vi "Save Patterns to Library.vi"(8 "error in (no error)":errorcluster, 11 "MultiPattern Matcher in":refnum<class "MultiPattern Matcher.lvclass">) -> (0 "error out":errorcluster, 3 "MultiPattern Matcher out":refnum<class "MultiPattern Matcher.lvclass">)   [LabVIEW 2013, in "MultiPattern Matcher.lvclass"]
uses:
  MultiPattern Matcher.lvclass
  MultiPattern Matcher.lvclass/MultiPattern Matcher.ctl
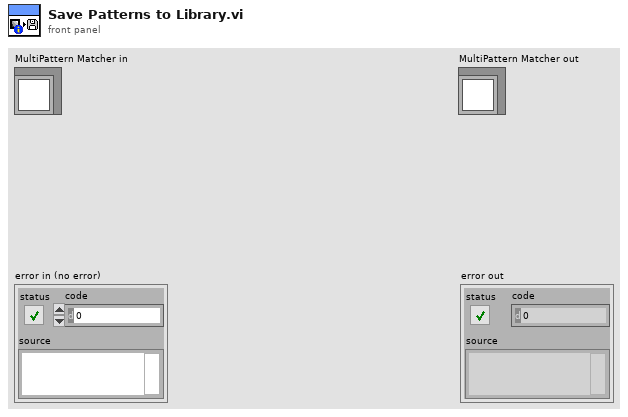
[diagram p1: front panel]
types:
  T1 = typedef "IMAQ Image.ctl" = refnum<image>
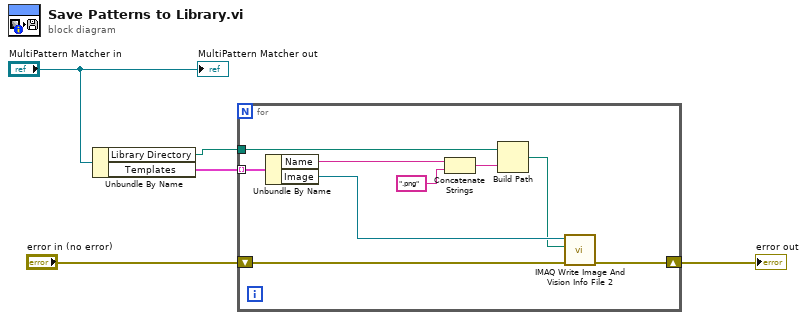
[diagram p0: block diagram]
diagram:
  n1 = Unbundle By Name("MultiPattern Matcher in") -> ("Library Directory"=w3:path, "Templates"=w4:cluster{"Image":T1, "Name":string}[])
  n2 = for {
    shift-right: [w6] -> w2
    shift-left: "error in (no error)" -> [w14]
    tunnel: w4 -> [w13] mode=indexing
    tunnel: w3 -> [w9]
    n3 = Unbundle By Name(w13) -> ("Name"=w11:string, "Image"=w8:T1)
    n4 = Concatenate Strings(w11, ".png" ("string")) -> (w10:string)
    n5 = Build Path(base path=w9, name or relative path=w10) -> (appended path=w7:path)
    n6 = call "IMAQ Write Image And Vision Info File 2"("error in (no error)"=w14, "File Path"=w7, "Image"=w8) -> ("error out"=w6:errorcluster)  [unwired: 7 in, 1 out]
  }
  "error out" <- w2
  "MultiPattern Matcher out" <- "MultiPattern Matcher in"
